vi "Websocket_Init.vi"(0 "reference in":refnum<class "Websocket.lvclass"> caption="This control should only be used when\na sub class is inheriting this class", 1 "websocket port (81)":u16=81, 5 "error in (no error)":errorcluster) -> (14 "reference out":refnum<class "Websocket.lvclass"> caption="This indicator should only be used when\na sub class is inheriting this class", 19 "error out":errorcluster)   [LabVIEW 2014, in "FrontPanelPublisher.lvlib" / "Websocket.lvclass"]
uses:
  Websocket.lvclass
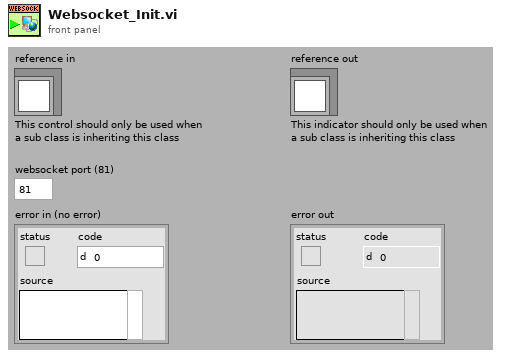
[diagram p1: front panel]
types:
  T1 = typedef "FrontPanelPublisher.lvlib/Websocket.lvclass/ObjectAttributes.ctl" = cluster{"Port":u16, "TCP Refs":refnum<k5>[]}
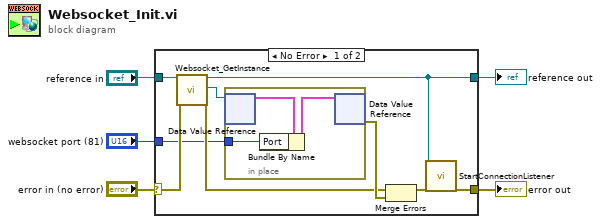
[diagram p0: block diagram]
diagram:
  n1 = case shown="No Error" "error in (no error)" {
    selector: "error in (no error)" -> [w11 w19]
    tunnel: [w6 w19] -> w4
    tunnel: "reference in" -> [w10 w18]
    tunnel: [w7 w18] -> w2
    tunnel: "websocket port (81)" -> [w8 _]
    frame No Error {
      n2 = call "Websocket_GetInstance.vi"("reference in"=w10, "error in (no error)"=w11) -> ("reference out"=w7:refnum<class "Websocket.lvclass">, "DVRRefOut"=w9:refnum<data-value>, "error out"=w13:errorcluster)  [unwired: 13 in, 2 out]
      n3 = in-place {
        in-place-border: w8 -> [w15]
        n4 = in-place-dvr #1(w9) -> (w16:T1)  [unwired: 1 out]
        n5 = Bundle By Name(cluster=w16, "Port"=w15) -> (w17:T1)
        n6 = in-place-dvr #1(w17) -> (w14:errorcluster)  [unwired: 1 out]
      }
      n7 = Merge Errors(w13, w14) -> (w12:errorcluster)
      n8 = call "StartConnectionListener.vi"("reference in"=w7, "error in (no error)"=w12) -> ("error out"=w6:errorcluster)  [unwired: 16 in, 1 out]
    }
    frame Error {
    }
  }
  "error out" <- w4
  "reference out" <- w2
